vi "Move Selected Layers.vi"(8 "error in":errorcluster, 10 "VKey":T8, 11 "Data in":T1={"Class"={"Ants"=refnum, "Layer"=refnum, "Templates"=refnum, "Icon"=refnum, "Glyph"=refnum, "Settings"=refnum, "Tools"=refnum}, "Ref"={"Add Layer"=refnum, "Remove Layer"=refnum, "Line Text"=[], "Body Text Spec"=refnum, "DNL_Font"=refnum, "glyph path str"=refnum, "templates path str"=refnum, "Arrow Up"=refnum, "Arrow Down"=refnum, "IE VI Ref"=refnum, "Glyphs tree"=refnum, "Templates tree"=refnum, "Layer Icon Text"=refnum, "Layer Template"=refnum, "Body Text"=refnum, "Search Templates"=refnum, "TextMarker"=refnum, "Tab Control"=refnum, "Search Glyphs"=refnum, "Line Color"=refnum, "DNL_Glyphs []"=refnum, "Fill Color"=refnum, "Tools"=refnum, "Icon"=refnum, "Preview"=refnum, "Ants"=refnum, "Terminals"=refnum, "menu reference"=refnum, "LayerNames"=[], "GlyphLoadAnimation"=refnum, "TemplateLoadAnimation"=refnum, "refreshGlyphs"=refnum, "refreshTemplates"=refnum}, "Support"={"AntsRect"={"left"=0, "top"=0, "right"=0, "bottom"=0}, "Mouse Move Coords"={"Horizontal"=0, "Vertical"=0}, "Mouse Down Coords"={"Horizontal"=0, "Vertical"=0}, "Temp Coord"={"Horizontal"=0, "Vertical"=0}, "Action"=enum."Default", "Edge Color"=4914962, "Fill Color"=16860, "Mouse Down?"=FALSE, "Draft Mode?"=FALSE, "Temp Icon"=bytes[3102], "CTRL Pressed"=FALSE, "Move Selection?"=FALSE, "AntsRect Orig"={"left"=0, "top"=0, "right"=0, "bottom"=0}, "Text"="", "TM Set?"=FALSE, "Mouse inside icon?"=FALSE, "Tool (old value)"=0, "Pencil Move Color"=0, "Swap Colors?"=FALSE, "Shift pressed?"=FALSE}}) -> (0 "error out":errorcluster, 3 "Data out":T1={"Class"={"Ants"=refnum, "Layer"=refnum, "Templates"=refnum, "Icon"=refnum, "Glyph"=refnum, "Settings"=refnum, "Tools"=refnum}, "Ref"={"Add Layer"=refnum, "Remove Layer"=refnum, "Line Text"=[], "Body Text Spec"=refnum, "DNL_Font"=refnum, "glyph path str"=refnum, "templates path str"=refnum, "Arrow Up"=refnum, "Arrow Down"=refnum, "IE VI Ref"=refnum, "Glyphs tree"=refnum, "Templates tree"=refnum, "Layer Icon Text"=refnum, "Layer Template"=refnum, "Body Text"=refnum, "Search Templates"=refnum, "TextMarker"=refnum, "Tab Control"=refnum, "Search Glyphs"=refnum, "Line Color"=refnum, "DNL_Glyphs []"=refnum, "Fill Color"=refnum, "Tools"=refnum, "Icon"=refnum, "Preview"=refnum, "Ants"=refnum, "Terminals"=refnum, "menu reference"=refnum, "LayerNames"=[], "GlyphLoadAnimation"=refnum, "TemplateLoadAnimation"=refnum, "refreshGlyphs"=refnum, "refreshTemplates"=refnum}, "Support"={"AntsRect"={"left"=0, "top"=0, "right"=0, "bottom"=0}, "Mouse Move Coords"={"Horizontal"=0, "Vertical"=0}, "Mouse Down Coords"={"Horizontal"=0, "Vertical"=0}, "Temp Coord"={"Horizontal"=0, "Vertical"=0}, "Action"=enum."Default", "Edge Color"=4914962, "Fill Color"=16860, "Mouse Down?"=FALSE, "Draft Mode?"=FALSE, "Temp Icon"=bytes[3102], "CTRL Pressed"=FALSE, "Move Selection?"=FALSE, "AntsRect Orig"={"left"=0, "top"=0, "right"=0, "bottom"=0}, "Text"="", "TM Set?"=FALSE, "Mouse inside icon?"=FALSE, "Tool (old value)"=0, "Pencil Move Color"=0, "Swap Colors?"=FALSE, "Shift pressed?"=FALSE}})   [LabVIEW 2020]
uses:
  Class/FakedArray/FakedArray.lvclass
  vi.lib/LabVIEW Icon API/lv_icon/Classes/Layer/Layer.lvclass
  <vilib>/Utility/miscctls.llb/LVPoint32TypeDef.ctl
  vi.lib/LabVIEW Icon API/lv_icon/Classes/Icon/Icon.lvclass
  <vilib>/event_ctls.llb/eventvkey.ctl
  Controls/SupportClass_Action.ctl
  vi.lib/LabVIEW Icon API/lv_icon/Controls/IEColor.ctl
  Controls/SupportClass.ctl
  Controls/References Cluster.ctl
  vi.lib/LabVIEW Icon API/lv_icon/lv_icon.lvlib
  Class/Tools/Tools Paint.lvclass
  Class/Settings/Settings.lvclass
  Class/Icon Library/Glyph.lvclass
  Class/Ants/Ants.lvclass
  Controls/IE Classes.ctl
  Controls/Global Data.ctl
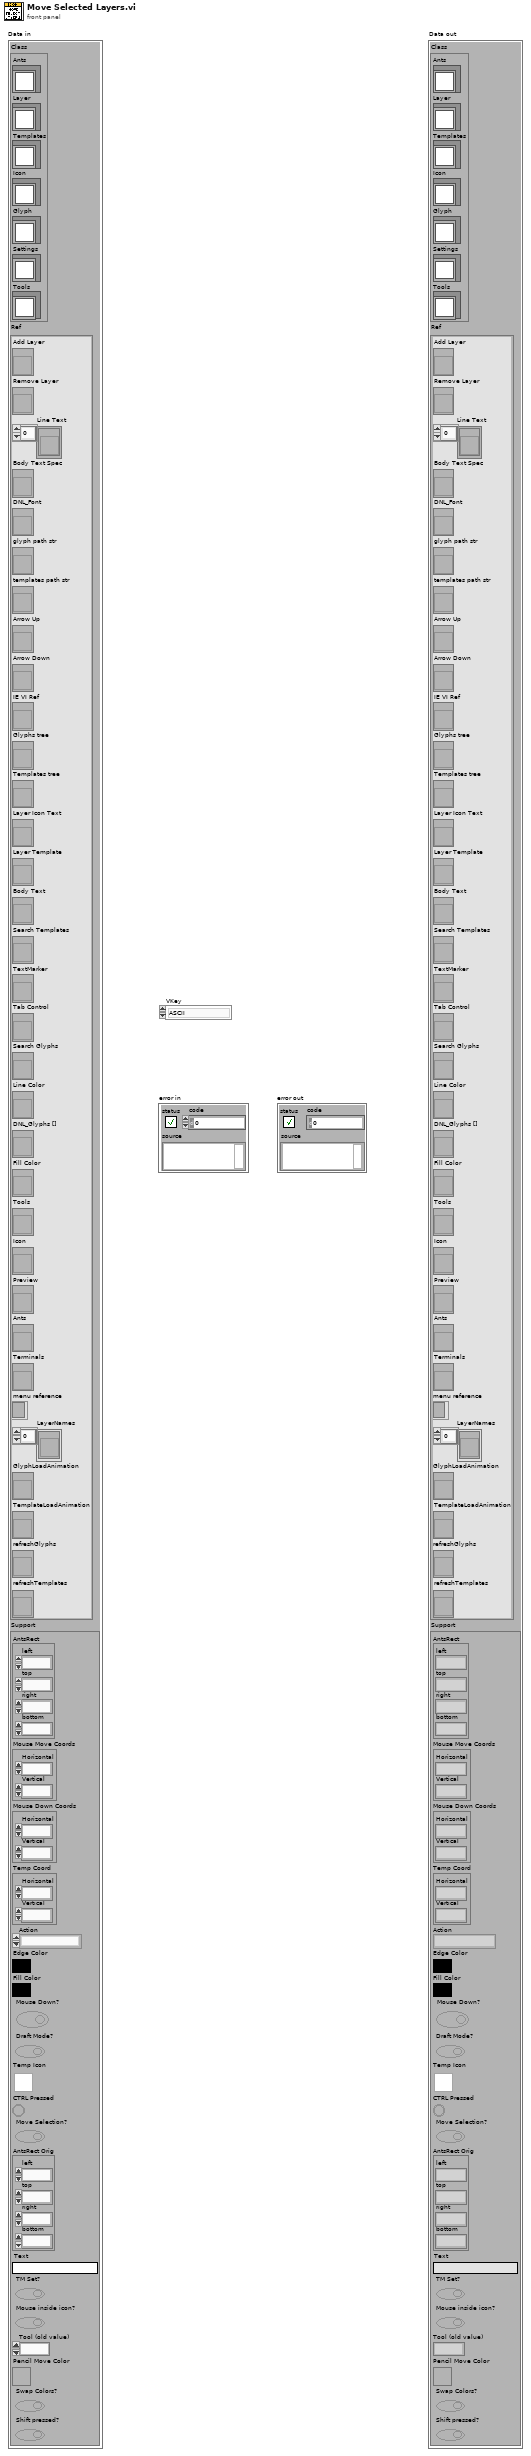
[diagram p1: front panel]
types:
  T1 = typedef "lv_icon.lvlib/Global Data.ctl" = cluster{"Class":T2, "Ref":T3, "Support":T4}
  T2 = typedef "IE Classes.ctl" = cluster{"Ants":refnum<class "Ants.lvclass">, "Layer":refnum<class "FakedArray.lvclass">, "Templates":refnum<class "FakedArray.lvclass">, "Icon":refnum<class "Icon.lvclass">, "Glyph":refnum<class "Glyph.lvclass">, "Settings":refnum<class "Settings.lvclass">, "Tools":refnum<class "Tools Paint.lvclass">}
  T3 = typedef "lv_icon.lvlib/References Cluster.ctl" = cluster{"Add Layer":refnum<vi>, "Remove Layer":refnum<vi>, "Line Text":refnum<vi>[], "Body Text Spec":refnum<vi>, "DNL_Font":refnum<vi>, "glyph path str":refnum<vi>, "templates path str":refnum<vi>, "Arrow Up":refnum<vi>, "Arrow Down":refnum<vi>, "IE VI Ref":refnum<vi>, "Glyphs tree":refnum<vi>, "Templates tree":refnum<vi>, "Layer Icon Text":refnum<vi>, "Layer Template":refnum<vi>, "Body Text":refnum<vi>, "Search Templates":refnum<vi>, "TextMarker":refnum<vi>, "Tab Control":refnum<vi>, "Search Glyphs":refnum<vi>, "Line Color":refnum<vi>, "DNL_Glyphs []":refnum<vi>, "Fill Color":refnum<vi>, "Tools":refnum<vi>, "Icon":refnum<vi>, "Preview":refnum<vi>, "Ants":refnum<vi>, "Terminals":refnum<vi>, "menu reference":refnum<k9>, "LayerNames":refnum<vi>[], "GlyphLoadAnimation":refnum<vi>, "TemplateLoadAnimation":refnum<vi>, "refreshGlyphs":refnum<vi>, "refreshTemplates":refnum<vi>}
  T4 = typedef "SupportClass.ctl" = cluster{"AntsRect":cluster{"left":i16, "top":i16, "right":i16, "bottom":i16}, "Mouse Move Coords":T5, "Mouse Down Coords":T5, "Temp Coord":T5, "Action":T6, "Edge Color":T7, "Fill Color":T7, "Mouse Down?":bool, "Draft Mode?":bool, "Temp Icon":picture, "CTRL Pressed":bool, "Move Selection?":bool, "AntsRect Orig":cluster{"left":i16, "top":i16, "right":i16, "bottom":i16}, "Text":string, "TM Set?":bool, "Mouse inside icon?":bool, "Tool (old value)":u32, "Pencil Move Color":u32, "Swap Colors?":bool, "Shift pressed?":bool}
  T5 = typedef "LVPoint32TypeDef.ctl" = cluster{"Horizontal":i32, "Vertical":i32}
  T6 = typedef "SupportClass_Action.ctl" = enum16{"Default", "Move Selection", "Glyph Library", "Tool"}
  T7 = typedef "IEColor.ctl" = u32
  T8 = typedef "eventvkey.ctl" = enum16{"ASCII", "Enter", "Return", "Shift", "Ctrl", "Alt", "Cmd", "Opt", "Caps", "NumLock", "Clear", "Break", "Up", "Down", "Left", "Right", "Insert", "Delete", "Home", "End", "PageUp", "PageDown", "Escape", "Help", "Pause", "ScrollLock", "F1", "F2", "F3", "F4", "F5", "F6", "F7", "F8", "F9", "F10", "F11", "F12", "F13", "F14", "F15", "F16", "F17", "F18", "F19", "F20", "F21", "F22", "F23", "F24", "Play", "VolumeUp", "VolumeDown", "Mute", "Two Byte Char"}
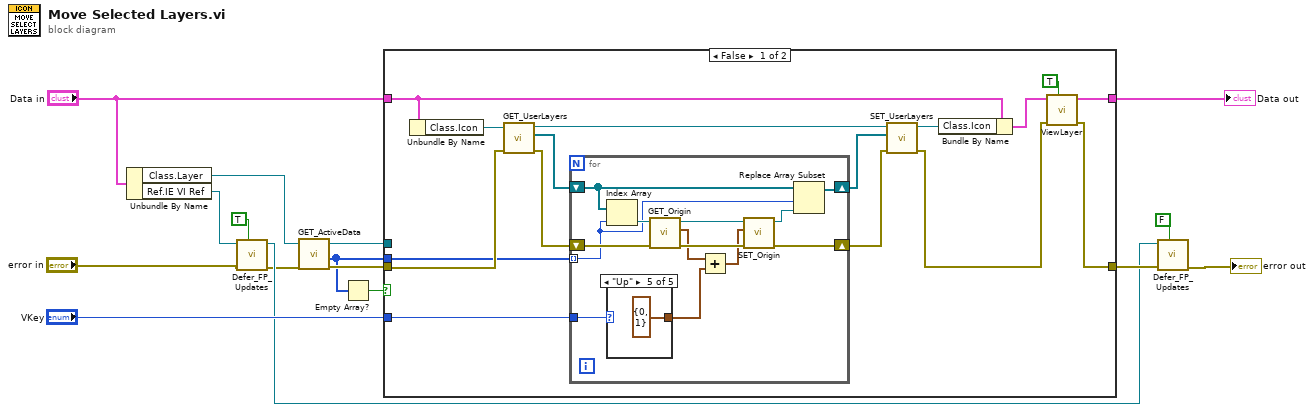
[diagram p0: block diagram]
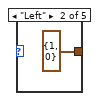
[diagram p3: hidden frame]
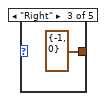
[diagram p4: hidden frame]
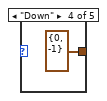
[diagram p5: hidden frame]
diagram:
  n1 = Unbundle By Name("Data in") -> ("Class.Layer"=w2:refnum<class "FakedArray.lvclass">, "Ref.IE VI Ref"=w3:refnum<vi>)
  n2 = call "Defer_FP_Updates.vi"("Defer Panel Updates"=TRUE, "error in"="error in", "lv_icon.vi in"=w3) -> ("error out"=w1:errorcluster, "lv icon.vi out"=w5:refnum<vi>)  [unwired: 7 out]
  n3 = call-dynamic "GET_ActiveData.vi"("error in (no error)"=w1, "FakedArray in"=w2) -> ("error out"=w9:errorcluster, "Active Data []"=w7:i32[], "FakedArray out"=w8:refnum<class "FakedArray.lvclass">)  [unwired: 7 out]
  n4 = Empty Array?(array=w7) -> (empty?=w10:bool)
  n5 = case shown="False" w10 {
    tunnel: [w18 w51] -> w6
    tunnel: w9 -> [w30 w51]
    tunnel: w8 -> [_ _]
    tunnel: w7 -> [w28 _]
    tunnel: "VKey" -> [w27 _]
    tunnel: "Data in" -> [w31 w50]
    tunnel: [w20 w50] -> w12
    frame False {
      n6 = Unbundle By Name(w31) -> ("Class.Icon"=w32:refnum<class "Icon.lvclass">)
      n7 = call-dynamic "GET_UserLayers.vi"("error in (no error)"=w30, "Icon.lvclass in"=w32) -> ("error out"=w26:errorcluster, "All Layers"=w29:refnum<class "Layer.lvclass">[], "Icon.lvclass out"=w25:refnum<class "Icon.lvclass">)  [unwired: 7 out]
      n8 = for {
        tunnel: w28 -> [w35] mode=indexing
        tunnel: w27 -> [w44]
        shift-right: [w33] -> w23
        shift-left: w26 -> [w43]
        shift-right: [w36] -> w24
        shift-left: w29 -> [w37]
        n9 = Index Array(array=w37, index=w35) -> (element=w45:refnum<class "Layer.lvclass">)
        n10 = case shown="\"Up\"" w44 {
          tunnel: [_ T5 {"Horizontal"=1, "Vertical"=0} ("Point32") T5 {"Horizontal"=-1, "Vertical"=0} ("Point32") T5 {"Horizontal"=0, "Vertical"=-1} ("Point32") T5 {"Horizontal"=0, "Vertical"=1} ("Point32")] -> w39
          frame "ASCII", Default {
          }
          frame "Left" {
          }
          frame "Right" {
          }
          frame "Down" {
          }
          frame "Up" {
          }
        }
        n11 = call-dynamic "GET_Origin.vi"("error in (no error)"=w43, "Layer.lvclass in"=w45) -> ("error out"=w41:errorcluster, "Point32"=w40:T5, "Layer.lvclass out"=w42:refnum<class "Layer.lvclass">)  [unwired: 7 out]
        n12 = Add(x=w40, y=w39) -> (x+y=w38:T5)
        n13 = call-dynamic "SET_Origin.vi"("error in"=w41, "Point32"=w38, "Layer.lvclass in"=w42) -> ("error out"=w33:errorcluster, "Layer.lvclass out"=w34:refnum<class "Layer.lvclass">)  [unwired: 7 out]
        n14 = Replace Array Subset(array=w37, new element=w34, index=w35) -> (w36:refnum<class "Layer.lvclass">[])
      }
      n15 = call-dynamic "SET_UserLayers.vi"("error in (no error)"=w23, "Layers"=w24, "Icon.lvclass in"=w25) -> ("error out"=w19:errorcluster, "Icon.lvclass out"=w22:refnum<class "Icon.lvclass">)  [unwired: 7 in]
      n16 = Bundle By Name(cluster=w31, "Class.Icon"=w22) -> (w21:T1)
      n17 = call "ViewLayer.vi"("Add to Undo?"=TRUE, "error in (no error)"=w19, "Data in"=w21) -> ("error out"=w18:errorcluster, "Data out"=w20:T1)  [unwired: 2 in, 5 out]
    }
    frame True {
    }
  }
  "Data out" <- w12
  n18 = call "Defer_FP_Updates.vi"("Defer Panel Updates"=FALSE, "error in"=w6, "lv_icon.vi in"=w5) -> ("error out"=→"error out":errorcluster)  [unwired: 8 out]
